vi "Configure Channel.vi"(0 "VISA resource name":refnum<visa-resource-name>, 1 "Enable Channel (T:Enable)":bool=TRUE, 5 "Channel (1: Channel 1)":u16(ring)=1 items=["Channel 1"=1, "Channel 2"=2, "Channel 3"=3, "Channel 4"=4], 7 "Vertical Coupling (0: DC)":u16(ring) items=["DC", "AC", "Ground"], 9 "Probe Attenuation (1.0)":dbl=1.0, 11 "error in (no error)":errorcluster, 12 "Vertical Range (1.0 V)":dbl=1.0, 13 "Vertical Offset (0.0 V)":dbl) -> (4 "VISA resource name out":refnum<visa-resource-name>, 15 "error out":errorcluster)   [LabVIEW 2025, in "RIGOL MHO900 Series.lvlib"]
uses:
  RIGOL MHO900 Series.lvlib
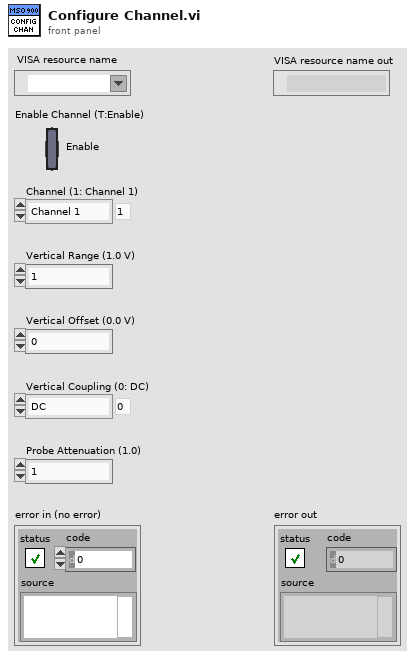
[diagram p1: front panel]
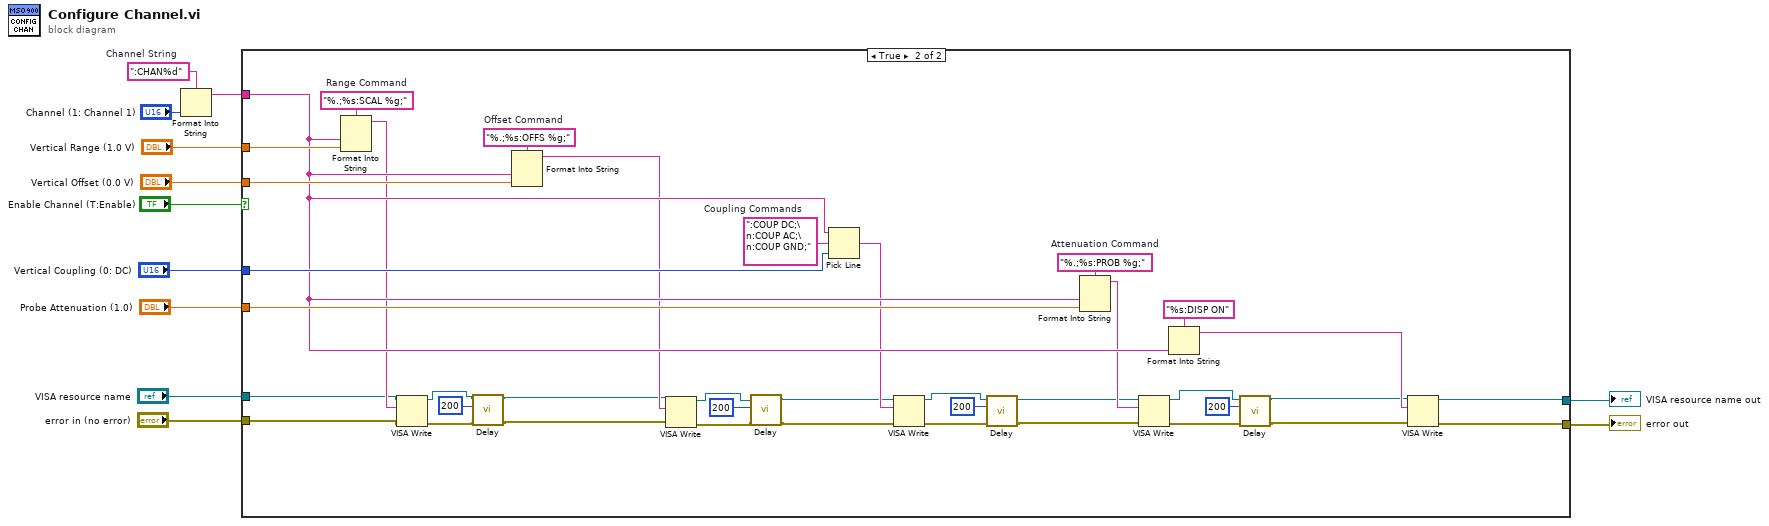
[diagram p0: block diagram]
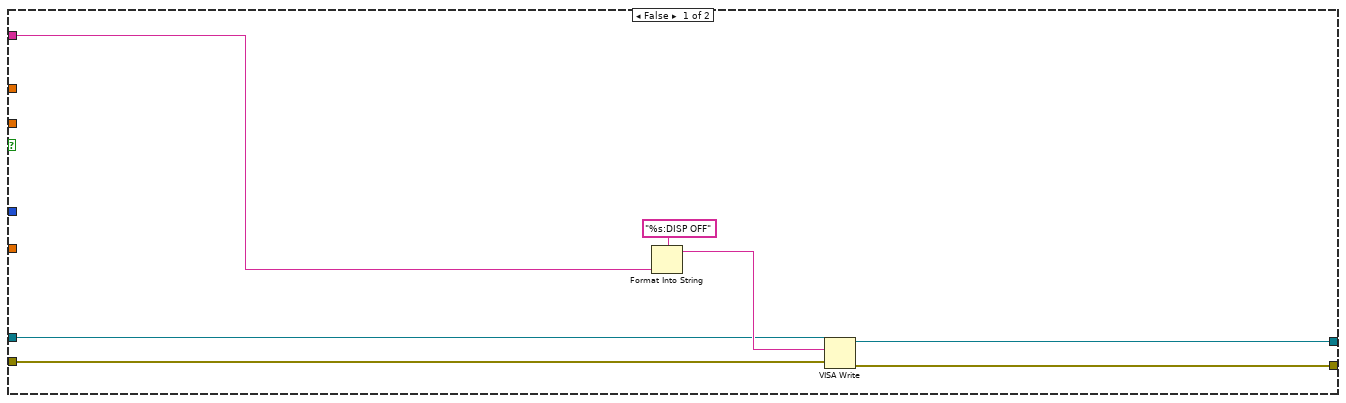
[diagram p2: hidden frame]
diagram:
  w10 = ":CHAN%d"  # Channel String
  n1 = Format Into String(format string=w10, "Channel (1: Channel 1)") -> (resulting string=w9:string)  [unwired: 2 in, 1 out]
  n2 = case shown="True" "Enable Channel (T:Enable)" {
    tunnel: w9 -> [w18 w49]
    tunnel: "Vertical Range (1.0 V)" -> [_ w53]
    tunnel: "Vertical Offset (0.0 V)" -> [_ w52]
    tunnel: "Vertical Coupling (0: DC)" -> [_ w51]
    tunnel: "Probe Attenuation (1.0)" -> [_ w50]
    tunnel: [w13 w40] -> w3
    tunnel: [w14 w41] -> w4
    tunnel: "VISA resource name" -> [w16 w43]
    tunnel: "error in (no error)" -> [w15 w42]
    frame False {
      n3 = Format Into String(format string="%s:DISP OFF", w18) -> (resulting string=w17:string)  [unwired: 2 in, 1 out]
      n4 = VISA Write(VISA resource name=w16, write buffer=w17, error in (no error)=w15) -> (VISA resource name out=w14:refnum<visa-resource-name>, error out=w13:errorcluster)  [unwired: 1 out]
    }
    frame True {
      w55 = "%.;%s:PROB %g;"  # Attenuation Command
      w56 = "%.;%s:SCAL %g;"  # Range Command
      w57 = "%.;%s:OFFS %g;"  # Offset Command
      w58 = ":COUP DC;\n:COUP AC;\n:COUP GND;"  # Coupling Commands
      n5 = Format Into String(format string=w56, w49, w53) -> (resulting string=w48:string)  [unwired: 2 in, 1 out]
      n6 = VISA Write(VISA resource name=w43, write buffer=w48, error in (no error)=w42) -> (VISA resource name out=w21:refnum<visa-resource-name>, error out=w24:errorcluster)  [unwired: 1 out]
      n7 = call "Delay.vi"("error in (no error)"=w24, "Delay (ms)"=u32 200, "VISA resource name"=w21) -> ("error out"=w23:errorcluster, "VISA resource name out"=w22:refnum<visa-resource-name>)  [unwired: 7 in]
      n8 = Format Into String(format string=w57, w49, w52) -> (resulting string=w47:string)  [unwired: 2 in, 1 out]
      n9 = VISA Write(VISA resource name=w22, write buffer=w47, error in (no error)=w23) -> (VISA resource name out=w35:refnum<visa-resource-name>, error out=w38:errorcluster)  [unwired: 1 out]
      n10 = call "Delay.vi"("error in (no error)"=w38, "Delay (ms)"=u32 200, "VISA resource name"=w35) -> ("error out"=w36:errorcluster, "VISA resource name out"=w37:refnum<visa-resource-name>)  [unwired: 7 in]
      n11 = Pick Line(string ("")=w49, multi-line string=w58, line index=w51) -> (output string=w46:string)
      n12 = VISA Write(VISA resource name=w37, write buffer=w46, error in (no error)=w36) -> (VISA resource name out=w30:refnum<visa-resource-name>, error out=w33:errorcluster)  [unwired: 1 out]
      n13 = call "Delay.vi"("error in (no error)"=w33, "Delay (ms)"=u32 200, "VISA resource name"=w30) -> ("error out"=w32:errorcluster, "VISA resource name out"=w31:refnum<visa-resource-name>)  [unwired: 7 in]
      n14 = Format Into String(format string=w55, w49, w50) -> (resulting string=w45:string)  [unwired: 2 in, 1 out]
      n15 = VISA Write(VISA resource name=w31, write buffer=w45, error in (no error)=w32) -> (VISA resource name out=w28:refnum<visa-resource-name>, error out=w27:errorcluster)  [unwired: 1 out]
      n16 = Format Into String(format string="%s:DISP ON", w49) -> (resulting string=w44:string)  [unwired: 2 in, 1 out]
      n17 = call "Delay.vi"("error in (no error)"=w27, "Delay (ms)"=u32 200, "VISA resource name"=w28) -> ("error out"=w25:errorcluster, "VISA resource name out"=w26:refnum<visa-resource-name>)  [unwired: 7 in]
      n18 = VISA Write(VISA resource name=w26, write buffer=w44, error in (no error)=w25) -> (VISA resource name out=w41:refnum<visa-resource-name>, error out=w40:errorcluster)  [unwired: 1 out]
    }
  }
  "error out" <- w3
  "VISA resource name out" <- w4
